vi "IOV engine refnum from target address.vi"(11 "target address":string) -> (3 "reference out":refnum<k21>)   [LabVIEW 2017]
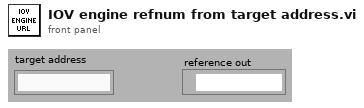
[diagram p1: front panel]
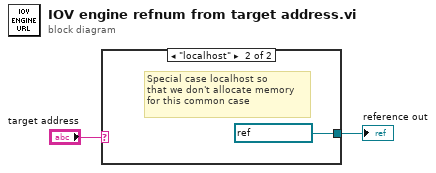
[diagram p0: block diagram]
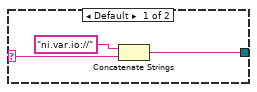
[diagram p2: hidden frame]
diagram:
  n1 = case shown="\"localhost\"" "target address" {
    selector: "target address" -> [w4 _]
    tunnel: [w3 refnum<k21> "ni.var.io:/" ("reference out")] -> w1
    frame Default {
      n2 = Concatenate Strings("ni.var.io://" ("string"), w4) -> (w3:string)
    }
    frame "localhost" {
      # "Special case localhost so\nthat we don't allocate memory\nfor this common case"
    }
  }
  "reference out" <- w1
